vi "Set Lock.vi"(8 "error in (no error)":errorcluster, 10 "Instrument Names":string[](array[string]), 11 "Sequence Context":refnum<k7>) -> (0 "error out":errorcluster, 2 "Status":i32[](array[numeric]), 3 "References":T1)   [LabVIEW 2019, in "Lock Library.lvlib"]
doc: "This VI locks a mutex, similar to TestStand's Lock step. It will attempt to lock a resource with every element in the Instrument Names array."
uses:
  Lock Library.lvlib
  References.ctl
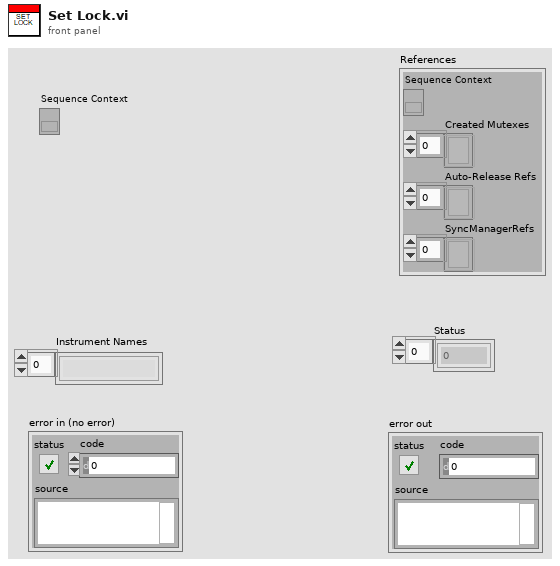
[diagram p1: front panel]
types:
  T1 = typedef "Lock Library.lvlib/References.ctl" = cluster{"Sequence Context":refnum<k7>, "Created Mutexes":refnum<k7>[], "Auto-Release Refs":refnum<k7>[], "SyncManagerRefs":refnum<k7>[]}
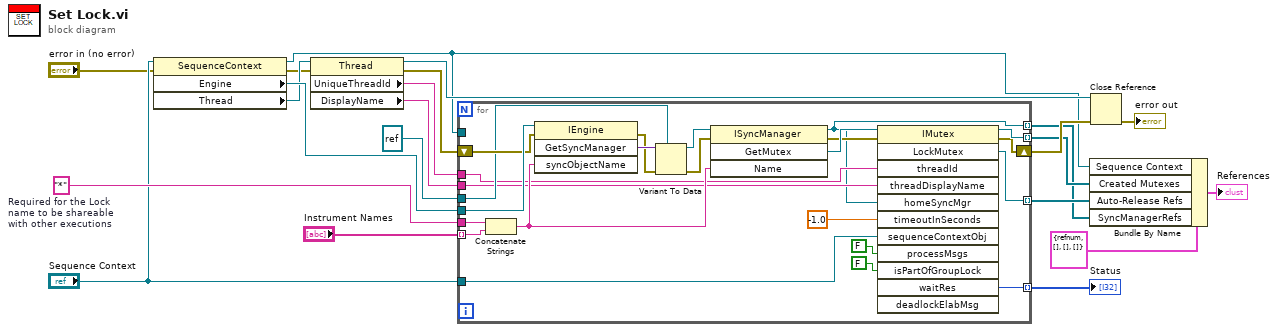
[diagram p0: block diagram]
diagram:
  w18 = "*"  # Required for the Lock name to be shareable with other executions
  n1 = property class="SequenceContext"(reference="Sequence Context", error in="error in (no error)") -> (reference out=w5:refnum<k7>, error out=w15:errorcluster, "Engine"=w21:refnum<k7>, "Thread"=w17:refnum<k7>)
  n2 = property class="Thread"(reference=w17, error in=w15) -> (reference out=w7:refnum<k7>, error out=w14:errorcluster, "UniqueThreadId"=w16:string, "DisplayName"=w13:string)
  n3 = for {
    tunnel: w21 -> [w44]
    tunnel: "Instrument Names" -> [w38] mode=indexing
    tunnel: refnum<k7> refnum ("TSSyncLib.ISyncManager") -> [w41]
    tunnel: w18 -> [w34]
    tunnel: w16 -> [w25]
    tunnel: w13 -> [w32]
    tunnel: "Sequence Context" -> [w31]
    tunnel: [w28] -> w11 mode=indexing
    tunnel: [w26] -> w4 mode=indexing
    shift-right: [w24] -> w9
    shift-left: w14 -> [w43]
    tunnel: w5 -> [_]
    tunnel: [w23] -> w3 mode=indexing
    tunnel: [w22] -> w2 mode=indexing
    n4 = Concatenate Strings(w34, w38) -> (w35:string)
    n5 = invoke class="IEngine" method="GetSyncManager"(reference=w44, error in=w43, "syncObjectName"=w35) -> (error out=w40:errorcluster, "GetSyncManager"=w42:variant)  [unwired: 1 in, 2 out]
    n6 = Variant To Data(error in=w40, type=w41, Variant=w42) -> (data=w39:refnum<k7>, error out=w37:errorcluster)
    n7 = invoke class="ISyncManager" method="GetMutex"(reference=w39, error in=w37, "Name"=w35) -> (reference out=w22:refnum<k7>, error out=w27:errorcluster, "GetMutex"=w36:refnum<k7>)  [unwired: 1 in, 1 out]
    n8 = invoke class="IMutex" method="LockMutex"(reference=w36, error in=w27, "threadId"=w25, "threadDisplayName"=w32, "homeSyncMgr"=w22, "timeoutInSeconds"=-1.0, "sequenceContextObj"=w31, "processMsgs"=FALSE, "isPartOfGroupLock"=FALSE) -> (reference out=w26:refnum<k7>, error out=w24:errorcluster, "LockMutex"=w23:refnum<k7>, "waitRes"=w28:i32)  [unwired: 3 in, 8 out]
  }
  "Status" <- w11
  n9 = Bundle By Name(cluster=T1 {"Sequence Context"=refnum, "Created Mutexes"=[], "Auto-Release Refs"=[], "SyncManagerRefs"=[]} ("References"), "Sequence Context"=w5, "Created Mutexes"=w4, "Auto-Release Refs"=w3, "SyncManagerRefs"=w2) -> (→"References":T1)
  n10 = Close Reference(reference=w7, error in (no error)=w9) -> (error out=→"error out":errorcluster)
